vi "Spectral Contrast.vi"(0 "Array":dbl[](array[numeric])) -> (1 "Sub_Band Valley":dbl[](array[numeric]), 2 "Sub-Band Peak":dbl[](array[numeric]), 3 "Sub-Band Average":dbl[](array[numeric]))   [LabVIEW 2013]
uses:
  <vilib>/Analysis/baseanly.llb/Mean (DBL).vi
  <vilib>/Analysis/NI_AALBase.lvlib
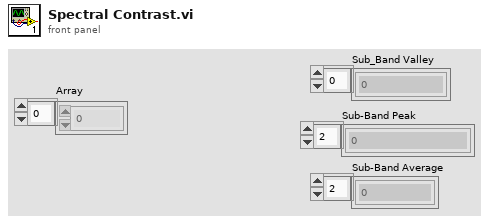
[diagram p1: front panel]
types:
  T1 = cluster{"1":dbl[], "2":dbl[], "3":dbl[], "4":dbl[], "5":dbl[], "6":dbl[], "7":dbl[]}
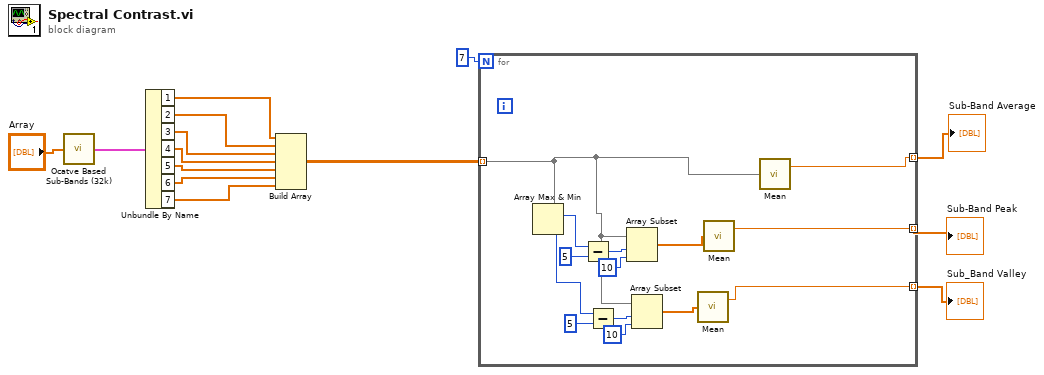
[diagram p0: block diagram]
diagram:
  n1 = call "Ocatve Based Sub-Bands (32k).vi"("Array"="Array") -> ("Sub-Band's"=w9:T1)
  n2 = Unbundle By Name(w9) -> ("1"=w8:dbl[], "2"=w7:dbl[], "3"=w6:dbl[], "4"=w5:dbl[], "5"=w4:dbl[], "6"=w3:dbl[], "7"=w2:dbl[])
  n3 = Build Array(w8, w7, w6, w5, w4, w3, w2) -> (w1:dbl[][])
  n4 = for {
    N: 7 -> [_]
    tunnel: [w24] -> w13 mode=indexing
    tunnel: [w22] -> w12 mode=indexing
    tunnel: [w16] -> w11 mode=indexing
    tunnel: w1 -> [w15] mode=indexing
    n5 = Array Max & Min(array=w15) -> (max index (indices)=w27:i32, min index (indices)=w18:i32)  [unwired: 2 out]
    n6 = Subtract(x=w27, y=5) -> (x-y=w28:i32)
    n7 = Subtract(x=w18, y=5) -> (x-y=w21:i32)
    n8 = Array Subset(array=w15, index=w28, length=10) -> (w23:dbl[])
    n9 = Array Subset(array=w15, index=w21, length=10) -> (w17:dbl[])
    n10 = call-poly <vilib>:"Mean.vi"("X"=w17) -> ("mean"=w16:dbl)  [unwired: 1 out]
    n11 = call-poly <vilib>:"Mean.vi"("X"=w23) -> ("mean"=w22:dbl)  [unwired: 1 out]
    n12 = call-poly <vilib>:"Mean.vi"("X"=w15) -> ("mean"=w24:dbl)  [unwired: 1 out]
  }
  "Sub-Band Average" <- w13
  "Sub-Band Peak" <- w12
  "Sub_Band Valley" <- w11
